vi "Write_Power_Off_Status.vi"(0 "Data File path":path, 5 "Value":bool=TRUE, 11 "error in (no error)":errorcluster) -> (15 "error out":errorcluster)   [LabVIEW 2020]
doc: "This VI writes the last time power off status done. Wheather normal shutdown or abort done"
uses:
  <vilib>/Utility/config.llb/Write Key (Boolean).vi
  <vilib>/Utility/config.llb/NI_LVConfig.lvlib
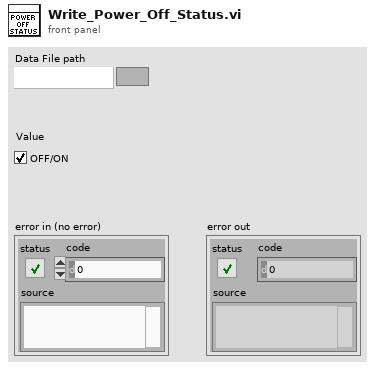
[diagram p1: front panel]
types:
  T1 = typedef "NI_LVConfig.lvlib/Config Data RefNum.ctl" = refnum<k1>
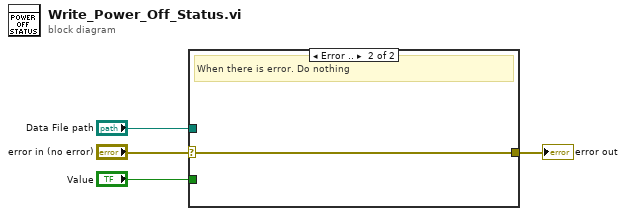
[diagram p0: block diagram]
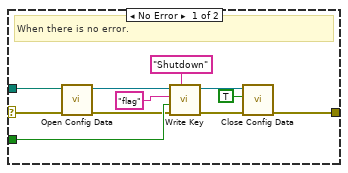
[diagram p2: hidden frame]
diagram:
  n1 = case shown="Error .." "error in (no error)" {
    selector: "error in (no error)" -> [w5 w16]
    tunnel: [w13 w16] -> w4
    tunnel: "Value" -> [w12 _]
    tunnel: "Data File path" -> [w7 _]
    frame No Error {
      # "When there is no error."
      n2 = call <vilib>:"Open Config Data.vi"("error in (no error)"=w5, "configuration file path"=w7) -> ("error out"=w6:errorcluster, "refnum"=w9:T1)  [unwired: 7 in, 1 out]
      n3 = call-poly <vilib>:"Write Key.vi"("section"="Shutdown", "error in (no error)"=w6, "value"=w12, "key"="flag", "refnum"=w9) -> ("error out"=w8:errorcluster, "refnum out"=w14:T1)  [unwired: 4 in, 1 out]
      n4 = call <vilib>:"Close Config Data.vi"("error in (no error)"=w8, "write file if changed (T)"=TRUE, "refnum"=w14) -> ("error out"=w13:errorcluster)  [unwired: 7 in, 1 out]
    }
    frame Error {
      # "When there is error. Do nothing"
    }
  }
  "error out" <- w4
